vi "Connect.vi"(8 "error in (no error)":errorcluster, 9 "coupler selection":T1, 10 "incident selection":T2, 11 "FPT_SParam_Switching in":refnum<class "FPT_SParam_Switching.lvclass">) -> (0 "error out":errorcluster, 3 "FPT_SParam_Switching out":refnum<class "FPT_SParam_Switching.lvclass">)   [LabVIEW 2023, in "FPT_SParam_Switching.lvclass"]
uses:
  FPT_SParam_Switching.lvclass
  <vilib>/niSPML/Switching/2 Couplers Per Port 1 VST/Incident Selection.ctl
  <vilib>/niSPML/Switching/2 Couplers Per Port 1 VST/Coupler Selection.ctl
  FPT_SParam_Switching.lvclass/FPT_SParam_Switching.ctl
  <vilib>/niSPML/Switching/2 Couplers Per Port 1 VST/S-Par 2 Couplers Per Port 1 VST Switching.lvclass
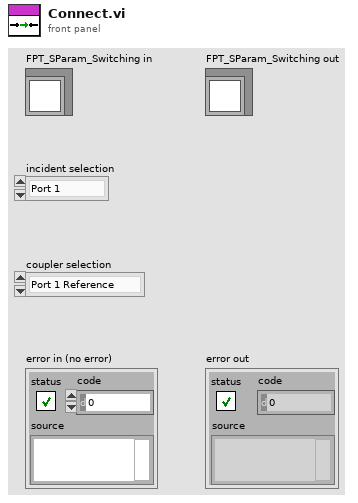
[diagram p1: front panel]
types:
  T1 = typedef "S-Par Switching.lvlib/S-Par 2 Couplers Per Port 1 VST Switching.lvclass/Coupler Selection.ctl" = enum16{"Port 1 Reference", "Port 1 Test", "Port 2 Reference", "Port 2 Test"}
  T2 = typedef "S-Par Switching.lvlib/S-Par 2 Couplers Per Port 1 VST Switching.lvclass/Incident Selection.ctl" = enum16{"Port 1", "Port 2"}
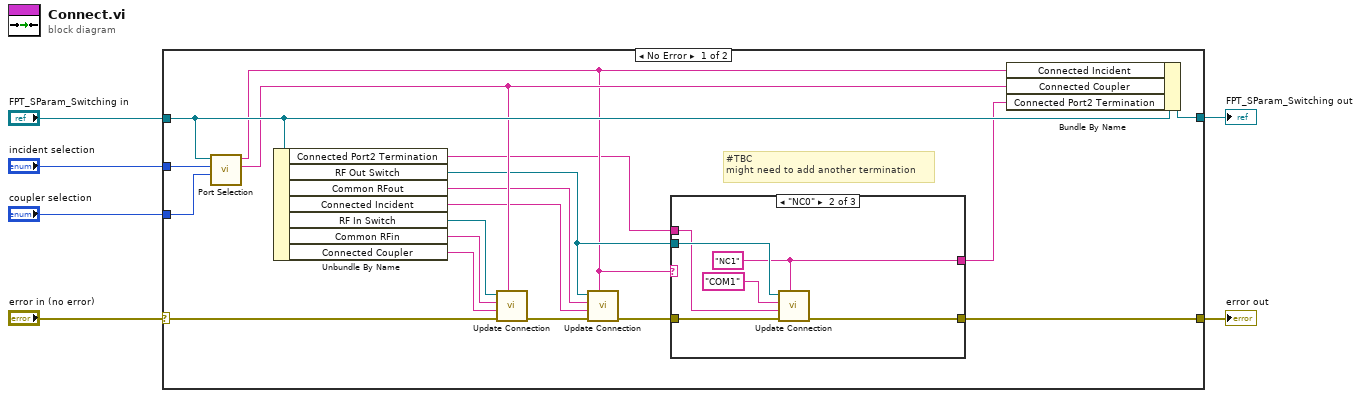
[diagram p0: block diagram]
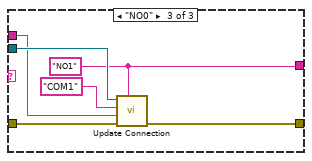
[diagram p3: hidden frame]
diagram:
  n1 = case shown="No Error" "error in (no error)" {
    selector: "error in (no error)" -> [w22 w39]
    tunnel: "incident selection" -> [w24 _]
    tunnel: "coupler selection" -> [w23 _]
    tunnel: "FPT_SParam_Switching in" -> [w18 w38]
    tunnel: [w12 w39] -> w2
    tunnel: [w14 w38] -> w1
    frame No Error {
      # "#TBC\nmight need to add another termination"
      n2 = call "Port Selection.vi"("Coupler Selection"=w23, "Incident Selection"=w24, "FPT_SParam_Switching in"=w18) -> ("Coupler Port"=w17:string, "Incident Port"=w10:string)  [unwired: 7 in]
      n3 = Unbundle By Name(w18) -> ("Connected Port2 Termination"=w7:string, "RF Out Switch"=w11:refnum<k15>, "Common RFout"=w15:string, "Connected Incident"=w9:string, "RF In Switch"=w19:refnum<k15>, "Common RFin"=w20:string, "Connected Coupler"=w21:string)
      n4 = call "Update Connection.vi"("new channel"=w17, "error in (no error)"=w22, "connected channel"=w21, "common channel"=w20, "switch"=w19) -> ("error out"=w16:errorcluster)  [unwired: 6 in]
      n5 = call "Update Connection.vi"("new channel"=w10, "error in (no error)"=w16, "connected channel"=w9, "common channel"=w15, "switch"=w11) -> ("error out"=w13:errorcluster)  [unwired: 6 in]
      n6 = case shown="\"NC0\"" w10 {
        tunnel: w13 -> [w25 w31 w37]
        tunnel: [w25 w30 w36] -> w12
        tunnel: w11 -> [_ w29 w35]
        tunnel: [_ w27 w33] -> w8
        tunnel: w7 -> [_ w26 w32]
        frame Default {
        }
        frame "NC0" {
          w27 = "NC1" ("connected channel")
          n7 = call "Update Connection.vi"("new channel"=w27, "error in (no error)"=w31, "connected channel"=w26, "common channel"="COM1", "switch"=w29) -> ("error out"=w30:errorcluster)  [unwired: 6 in]
        }
        frame "NO0" {
          w33 = "NO1" ("connected channel")
          n8 = call "Update Connection.vi"("new channel"=w33, "error in (no error)"=w37, "connected channel"=w32, "common channel"="COM1", "switch"=w35) -> ("error out"=w36:errorcluster)  [unwired: 6 in]
        }
      }
      n9 = Bundle By Name(cluster=w18, "Connected Incident"=w10, "Connected Coupler"=w17, "Connected Port2 Termination"=w8) -> (w14:refnum<class "FPT_SParam_Switching.lvclass">)
    }
    frame Error {
    }
  }
  "error out" <- w2
  "FPT_SParam_Switching out" <- w1
